vi "WINDOW-System Config.vi"() -> ()   [LabVIEW 2020]
uses:
  User Interface/Windows/System config window/Globals/Sys Config window globals.vi
  User Interface/Windows/System config window/Typedefs/HW config window refs cluster.ctl
  Global Variables/General Globals.vi
  Typedefs/HW config states enum.ctl
  Global Variables/gl_UI Ctrl Refs.vi
  User Interface/Visualisation/Functional Imaging Viewer/Typedefs/Get-Set-Clear Control.ctl
  <vilib>/userDefined/High Color/nirio_resource_hc.ctl
  Typedefs/FPGA input type AC-DC.ctl
  User Interface/Windows/System config window/Typedefs/HW Setup tab control.ctl
  Peripherals Control/Triggers/Typedefs/Trigger setup element cluster.ctl
  Peripherals Control/Triggers/Typedefs/Triggers output setup.ctl
  Typedefs/CTRL system config cluster.ctl
  Typedefs/AOL Properties Cluster.ctl
  RIG-SPECIFIC FILES/FPGA Refs/FPGA Ref.ctl
  Typedefs/DAQ FPGA config cluster.ctl
  Typedefs/Trigger 1 selector enum.ctl
  Peripherals Control/Triggers/Typedefs/General trigger settings cluster.ctl
  Typedefs/Laser 1 config cluster.ctl
  Typedefs/PreChirper 1 config cluster.ctl
  Typedefs/Encoder config cluster.ctl
  Typedefs/Laser Power Control HW config.ctl
  Typedefs/Cam VidRec HW config setup cluster.ctl
  Typedefs/Triggers HW config.ctl
  Typedefs/Objective Config.ctl
  Typedefs/AOD Settings-distilled.ctl
  Typedefs/Prechirper Cal Config.ctl
  Typedefs/PreChirper constants.ctl
  Typedefs/CTRL system config.ctl
  Typedefs/Control Sys HW config cluster.ctl
  Typedefs/DAQ FPGA HW config cluster.ctl
  Typedefs/DAQ FPGA system config.ctl
  Typedefs/Comms Type.ctl
  Typedefs/Peripherals comms config cluster.ctl
  Peripherals Control/XYZ Stage/Control/typedefs/XYZControlConfig.ctl
panel:
  in  "Y stage available":bool
  in  "Y Comms Config Cluster":T1
  in  "DAQ FPGA config cluster":T3={"Target"="RIO0", "input card type"=enum."AC Card", "Ref"=refnum, "Clock Freq (MHz) "=200.0, "Samples Wait after Trigger"=5080, "AOD fill"=4900, "StartupDelay"=0, "Slip Cycle (clock cycles)"=600000, "Add Cycle"=TRUE}
  in  "Control system":T7={"Contrl Sys Available Ind"=FALSE, "Control system.FPGA Type"=enum."Virtex 5", "Control system.Network adapter name"="", "Control system.MAC address"="", "Control system.Ethernet Port"=3, "Ethernet opened"=FALSE, "Ctrl FPGA Clock (MHz)"=240.0, "AOD 1 Amplitude"=0, "AOD 2 Amplitude"=0, "AOD 3 Amplitude"=0, "AOD 4 Amplitude"=0, "AOD 5 Amplitude"=0, "AOD 6 Amplitude"=0, "Data Time Interval (ns)"=0.0, "T0 (ns)"=0.0, "Ta (ns)"=0.0} {"Control system.Ethernet Port" min=0 max=2048 step=1; "Ctrl FPGA Clock (MHz)" min=80.0 max=500.0 step=1.0; "Data Time Interval (ns)" min=0.0 max=2048.0 step=1.0; "Ta (ns)" min=0.0 max=2048.0 step=1.0; "T0 (ns)" min=0.0 max=2048.0 step=1.0; "AOD 6 Amplitude" min=0 max=2048 step=1; "AOD 5 Amplitude" min=0 max=2048 step=1; "AOD 4 Amplitude" min=0 max=2048 step=1; "AOD 3 Amplitude" min=0 max=2048 step=1; "AOD 2 Amplitude" min=0 max=2048 step=1; "AOD 1 Amplitude" min=0 max=2048 step=1}
  in  "Cancel":bool
  in  "OK":bool
  in  "AOL Properties":T8={"AOD 1 thickness (mm)"=118.0, "AOD 2 thickness (mm)"=115.0, "AOD 3 thickness (mm)"=110.0, "AOD 4 thickness (mm)"=135.0, "AOD 5 thickness (mm)"=135.0, "AOD 6 thickness (mm)"=135.0, "AOD 1-2 separation (mm)"=15.0, "AOD 2-3 separation (mm)"=15.0, "AOD 3-4 separation (mm)"=15.0, "AOD 4-5 separation (mm)"=15.0, "AOD 5-6 separation (mm)"=15.0, "AOD 1 X Offset"=15.0, "AOD 2 X Offset"=1.0, "AOD 3 X Offset"=1.0, "AOD 4 X Offset"=1.0, "AOD 1 Y Offset"=1.0, "AOD 2 Y Offset"=1.0, "AOD 3 Y Offset"=1.0, "AOD 4 Y Offset"=1.0, "AOD 1 X Direction"=0.0, "AOD 2 X Direction"=0.0, "AOD 3 X Direction"=0.0, "AOD 4 X Direction"=0.0, "AOD 1 Y Direction"=1.0, "AOD 2 Y Direction"=0.0, "AOD 3 Y Direction"=0.0023, "AOD 4 Y Direction"=0.0046, "AOD 1 Centre (mm)"=15.0, "AOD 2 Centre (mm)"=50.0, "AOD 3 Centre (mm)"=50.0, "AOD 4 Centre (mm)"=50.0, "Timing Offset AOD 1"=0.0, "Timing Offset AOD 2"=0.0, "Timing Offset AOD 3"=0.0, "Timing Offset AOD 4"=0.0, "AOD Optical offset 1"=20000.0, "AOD Optical offset 2"=20000.0, "AOL aperture (mm)"=15.0, "AOL centre wavelength (nm)"=1.0, "AOL centre frequency (MHz)"=1.0, "Diffraction mode"=1.0, "Crystal length (mm)"=0.0, "Acoustic velocity (m/s)"=1.0, "Pair deflection ratio"=1.0, "AOD fill time (us)"=1.0, "AOD Ord. Refractive index"=2.22, "AOD ExtraOrd. Refractive index"=2.22}
  in  "Config Tab Control":T9=enum."Hardware Setup"
  in  "Control Sys. HW config":T10
  in  "Controller System Config":T11={"AOD 1 Amplitude"=0, "AOD 2 Amplitude"=0, "AOD 3 Amplitude"=0, "AOD 4 Amplitude"=0, "AOD 5 Amplitude"=0, "AOD 6 Amplitude"=0, "T0 (ns)"=0.0, "Ta (ns)"=0.0, "Data Time Interval (ns)"=0.0, "Ctrl FPGA Clock (MHz)"=240.0} {"Ctrl FPGA Clock (MHz)" min=80.0 max=500.0 step=1.0; "Data Time Interval (ns)" min=0.0 max=2048.0 step=1.0; "Ta (ns)" min=0.0 max=2048.0 step=1.0; "T0 (ns)" min=0.0 max=2048.0 step=1.0; "AOD 6 Amplitude" min=0 max=2048 step=1; "AOD 5 Amplitude" min=0 max=2048 step=1; "AOD 4 Amplitude" min=0 max=2048 step=1; "AOD 3 Amplitude" min=0 max=2048 step=1; "AOD 2 Amplitude" min=0 max=2048 step=1; "AOD 1 Amplitude" min=0 max=2048 step=1}
  in  "Ctrl FPGA available":bool
  in  "DAQ FPGA System Config":T12={"Clock Freq (MHz) "=200.0, "Samples Wait after Trigger"=5080, "AOD fill"=4900, "StartupDelay"=0, "Slip Cycle (clock cycles)"=600000, "Add Cycle"=TRUE}
  in  "DAQ FPGA HW Config":T13={"FGPA Ref"=refnum, "Target"="RIO0", "input card type"=enum."AC Card"}
  in  "Triggers sub-tab control":enum32{"General", "Routing & Timing"}(tab)
  in  "Trigger HW config":T14
  in  "General trigger settings":T15={"Trigger 1 function"=enum."Encoder trigger", "Triggers loop clock (MHz)"=80.0} {"Triggers loop clock (MHz)" format="%#_13g"}
  in  "Triggers output setup":T17 {"Pulse width (us)" min=10 max=5000 step=1 format="%.0fµs"}
  in  "Externalise Triggers":bool
  in  "PMT Voltage Upper Limit":dbl
  in  "PMT Voltage Lower Limit":dbl
  in  "Galvo AOs":tag
  in  "Power meter AI":tag
  in  "Pockels AO":tag
  in  "PMT AOs":tag
  in  "Hard shutter AO":tag
  in  "Z Comms Config Cluster":T1
  in  "XY Comms Config Cluster":T1
  in  "Z stage available":bool
  in  "XY stage available":bool
  in  "XYZ Stage Control Config":T19
  in  "Encoder":T20={"IP address"="224.0.1.103", "Port"=7000, "Wheel radius (cm)"=16.0, "Encoder Trigger"=""} {"Wheel radius (cm)" format="%#_13g"}
  in  "Wheel radius (cm)":dbl format="%#_13g"
  in  "Encoder IP address":string="224.0.1.103"
  in  "Encoder port":u16=7000
  in  "Encoder available":bool
  in  "Axial MC Supported":bool caption="Axial Movement Correction Supported"
  in  "MC Supported":bool caption="Movement Correction Supported"
  in  "Computer MAC address":string="82574L"
  in  "Demo mode":enum16{"Full functionality", "Demo mode"}(ring) caption="Mode"
  in  "Number of AODs":dbl=4.0
  in  "Swap XY on stage":bool
  in  "DO flag-Trial start":tag
  in  "DO flag-Video record":tag
  in  "Cam VidRec available":bool caption="Cameras video recording system is available"
  in  "Cam VidRec":T21
  in  "AOD Settings - distilled":T22={"AOD 1 thickness (mm)"=8.0, "AOD 2 thickness (mm)"=8.0, "AOD 3 thickness (mm)"=8.0, "AOD 4 thickness (mm)"=8.0, "AOD 1-2 separation (mm)"=50.0, "AOD 2-3 separation (mm)"=50.0, "AOD 3-4 separation (mm)"=50.0, "AOD 1 Centre (mm)"=7.5, "AOD 2 Centre (mm)"=7.5, "AOD 3 Centre (mm)"=7.5, "AOD 4 Centre (mm)"=7.5, "AOD 1 X Offset"=0.0, "AOD 2 X Offset"=0.0023, "AOD 3 X Offset"=0.0046, "AOD 4 X Offset"=0.0046, "AOD 1 Y Offset"=0.0, "AOD 2 Y Offset"=0.0, "AOD 3 Y Offset"=0.0023, "AOD 4 Y Offset"=0.0046, "Timing Offset AOD 1"=0.0, "Timing Offset AOD 2"=0.0, "Timing Offset AOD 3"=0.0, "Timing Offset AOD 4"=0.0, "AOL centre wavelength (nm)"=1.0, "AOL centre frequency (MHz)"=1.0, "Pair deflection ratio"=1.0, "AOL aperture (mm)"=15.0, "AOD fill time (us)"=1.0, "Diffraction mode"=1.0, "Crystal length (mm)"=0.0, "Acoustic velocity (m/s)"=1.0, "AOD Ord. Refractive index"=2.22}
  in  "Current Objective":string
  in  "Objective Calibration Settings":T23[](array[typedef])
  in  "Pockels cal.Dwell time (µs)":dbl=0.4 caption="Dwell time (µs)" min=0.05 max=12.0 step=0.1 format="%#.2fµs"
  in  "Pockels cal.Zoom":u8=12 caption="Zoom" min=1 max=24 step=1 format="x%.0f"
  in  "Laser 1 available":bool
  in  "Laser 1 config":T24={"COM port"="COM7", "Baud Rate"=0, "Type"=""}
  in  "Laser Power Control HW config":T25={"Laser Power Control"="Pockels", "Laser Power Modulation Control"=enum."NI"}
  in  "Laser Wavelength 2":u16(ring) caption="Laser Wavelength (nm)" items=["920"]
  in  "Prechirper 1 available":bool
  in  "Prechirper 1 config":T26={"Type"="", "Baud Rate"=0, "COM port"="COM7"}
  in  "PreChirper Preset Calibration Values":T27[](array[typedef])
  in  "Prechirper Constants":T28
  in  "PreChirp Preset Values":bool caption="Use Preset Values"
  in  "Initial Laser Wavelength [nm]":dbl=5.0
  in  "Initial Dwell Time [us]":dbl=5.0
  in  "Error Logging":bool
  in  "Performance Monitoring":bool caption="PC Performance Monitoring"
  in  "Microscope ID":string="003"
  in  "Microscope Type":string="AOLM"
  in  "Revision Number":string="1.0.0.0"
  in  "Advanced Imaging":bool
  in  "Max Allowed Trial Length [s]":dbl=60.0
  in  "Initial Scan Resolution":dbl=512.0
  in  "Initial Acceptance Angle [mrad]":dbl=5.0
  # "This functionality connects the various PXI backplane triggers to physical terminals on the DI/O module.\n\n\nOriginal setup:\nPXI_Trigger 0= Unused\nPXI_Trigger 1= Line trigger\nPXI_Trigger 2= Frame trigger / Cycle trigge\nPXI_Trigger 3= Trial trigger\nPXI_Trigger 4= Start of Experiment trigger\nPXI_Trigger 5= Stimulus trigger"
  # "(make , model etc)"
  # "(COM Port / IP Address / service address etc.)"
  # "(Port for ethernet / channel for BT)"
  # "[HWC]"
  # "[DNT]"
  # "NOTE: The triggers setup is part of the user-profiles functionality.\nSave the current user profile to retain any changes you make above.\nChanges will not be automatically saved."
  # "'Externalise Triggers' must be enabled"
  # "[DNT]"
  # "[HWC]"
  # "(make , model etc)"
  # "(COM Port / IP Address / service address etc.)"
  # "(Port for ethernet / channel for BT)"
  # "(make , model etc)"
  # "(COM Port / IP Address / service address etc.)"
  # "(Port for ethernet / channel for BT)"
  # "[Delete me later]"
  # "Thickness (mm)"
  # "X Offset"
  # "Separation (mm)"
  # "Y Offset"
  # "Centre (mm)"
  # "Timing Offset"
  # "Pockels Calibration Conditions"
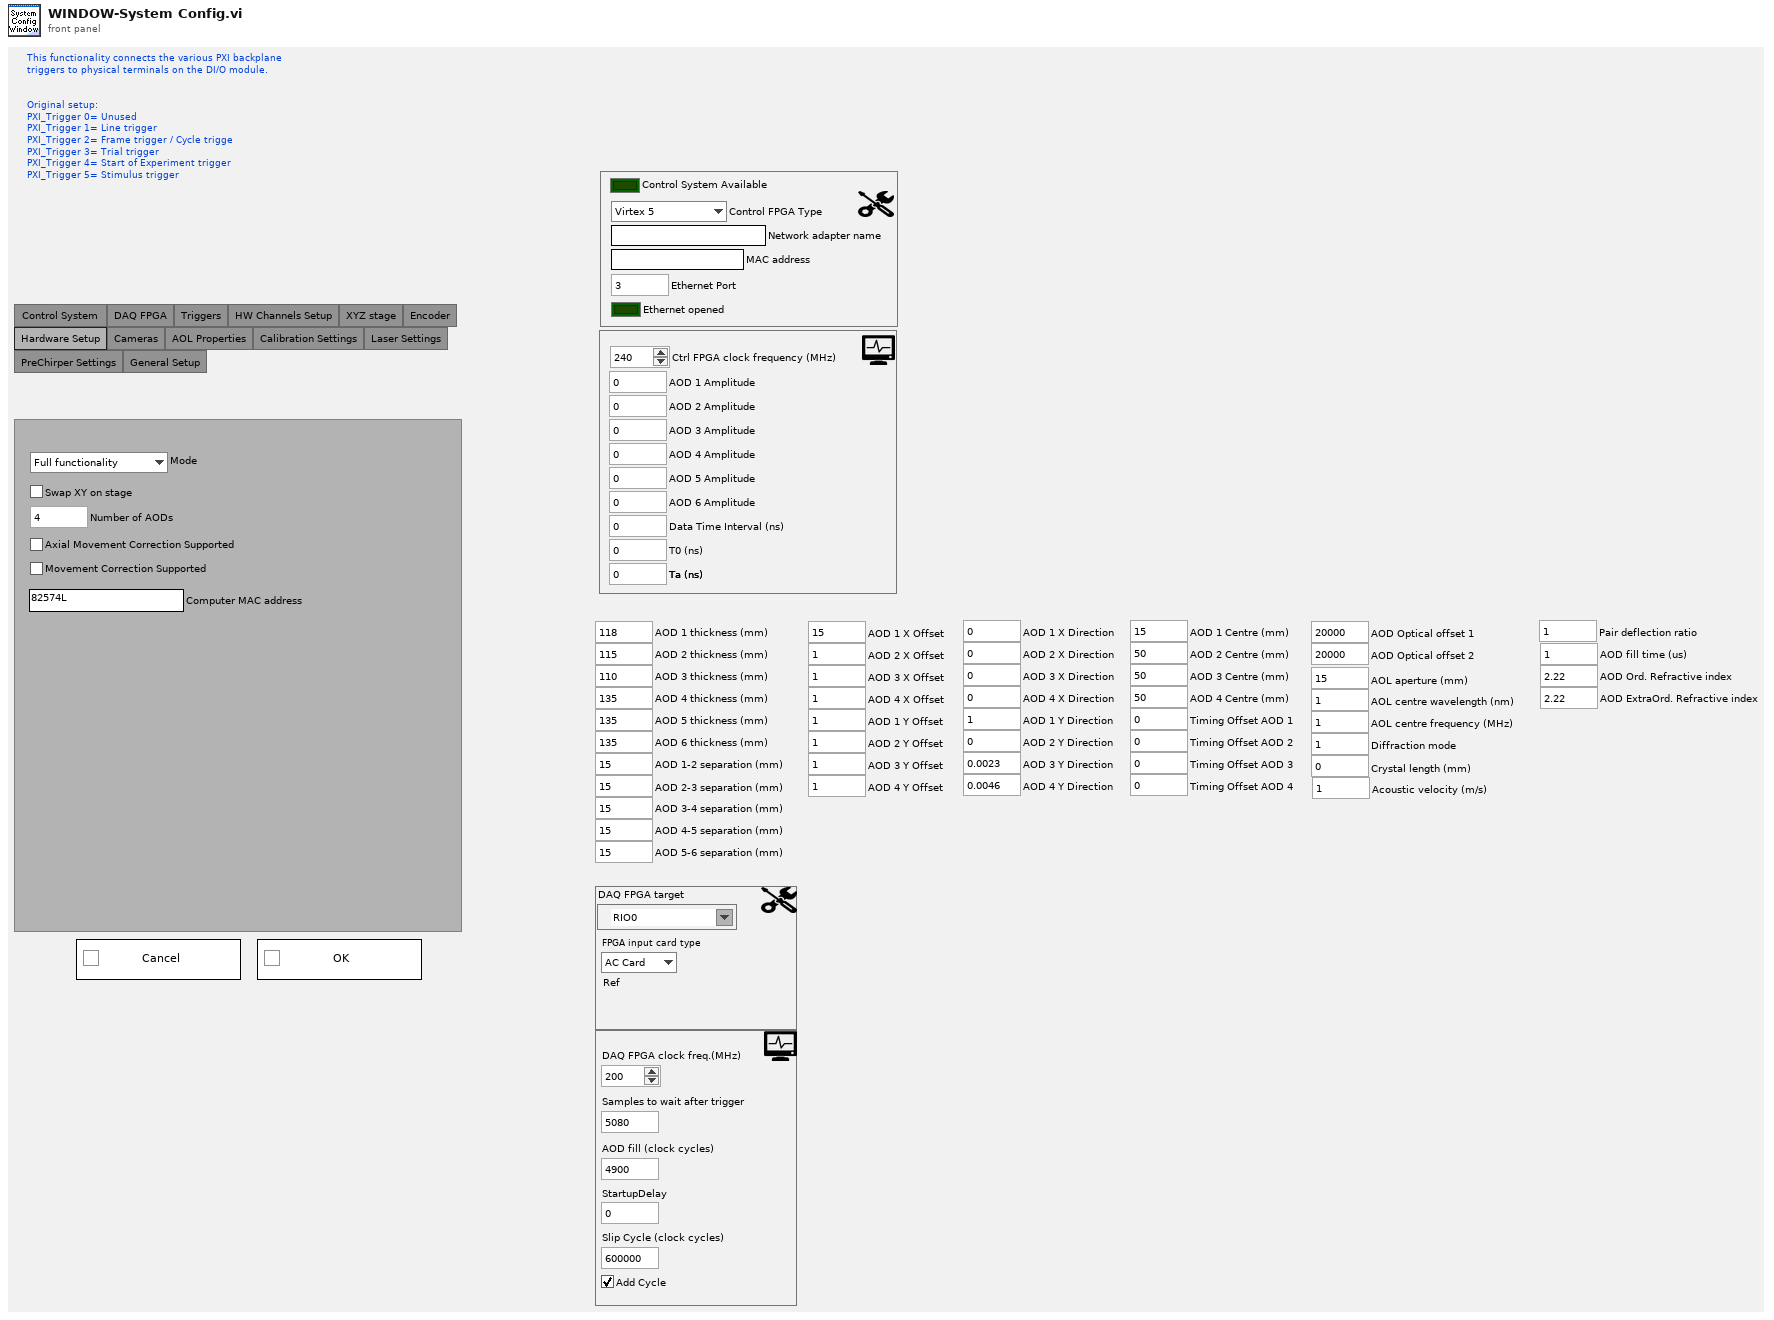
[diagram p1: front panel]
types:
  T1 = typedef "Peripherals comms config cluster.ctl" = cluster{"Name":string, "Device Address":string, "Port ":u16, "Baudrate":i32, "Comms Type":T2}
  T2 = typedef "Comms Type.ctl" = enum16{"GPIB-IEEE488", "Serial-RS232", "Serial-RS485", "Serial-RS422", "Serial-USB", "Ethernet-TCP/IP", "Ethernet-UDP"}
  T3 = typedef "DAQ FPGA config cluster.ctl" = cluster{"Target":T4, "input card type":T5, "Ref":T6, "Clock Freq (MHz) ":dbl, "Samples Wait after Trigger":u16, "AOD fill":u16, "StartupDelay":i32, "Slip Cycle (clock cycles)":u32, "Add Cycle":bool}
  T4 = typedef "nirio_resource_hc.ctl" = tag
  T5 = typedef "FPGA input type AC-DC.ctl" = enum16{"AC Card", "DC Card"}
  T6 = typedef "FPGA Ref.ctl" = refnum<k20>
  T7 = typedef "CTRL system config cluster.ctl" = cluster{"Contrl Sys Available Ind":bool, "Control system.FPGA Type":enum16{"Virtex 5", "Virtex 7"}, "Control system.Network adapter name":string, "Control system.MAC address":string, "Control system.Ethernet Port":i16, "Ethernet opened":bool, "Ctrl FPGA Clock (MHz)":dbl, "AOD 1 Amplitude":i16, "AOD 2 Amplitude":i16, "AOD 3 Amplitude":i16, "AOD 4 Amplitude":i16, "AOD 5 Amplitude":i16, "AOD 6 Amplitude":i16, "Data Time Interval (ns)":dbl, "T0 (ns)":dbl, "Ta (ns)":dbl}
  T8 = typedef "AOL Properties Cluster.ctl" = cluster{"AOD 1 thickness (mm)":dbl, "AOD 2 thickness (mm)":dbl, "AOD 3 thickness (mm)":dbl, "AOD 4 thickness (mm)":dbl, "AOD 5 thickness (mm)":dbl, "AOD 6 thickness (mm)":dbl, "AOD 1-2 separation (mm)":dbl, "AOD 2-3 separation (mm)":dbl, "AOD 3-4 separation (mm)":dbl, "AOD 4-5 separation (mm)":dbl, "AOD 5-6 separation (mm)":dbl, "AOD 1 X Offset":dbl, "AOD 2 X Offset":dbl, "AOD 3 X Offset":dbl, "AOD 4 X Offset":dbl, "AOD 1 Y Offset":dbl, "AOD 2 Y Offset":dbl, "AOD 3 Y Offset":dbl, "AOD 4 Y Offset":dbl, "AOD 1 X Direction":dbl, "AOD 2 X Direction":dbl, "AOD 3 X Direction":dbl, "AOD 4 X Direction":dbl, "AOD 1 Y Direction":dbl, "AOD 2 Y Direction":dbl, "AOD 3 Y Direction":dbl, "AOD 4 Y Direction":dbl, "AOD 1 Centre (mm)":dbl, "AOD 2 Centre (mm)":dbl, "AOD 3 Centre (mm)":dbl, "AOD 4 Centre (mm)":dbl, "Timing Offset AOD 1":dbl, "Timing Offset AOD 2":dbl, "Timing Offset AOD 3":dbl, "Timing Offset AOD 4":dbl, "AOD Optical offset 1":dbl, "AOD Optical offset 2":dbl, "AOL aperture (mm)":dbl, "AOL centre wavelength (nm)":dbl, "AOL centre frequency (MHz)":dbl, "Diffraction mode":dbl, "Crystal length (mm)":dbl, "Acoustic velocity (m/s)":dbl, "Pair deflection ratio":dbl, "AOD fill time (us)":dbl, "AOD Ord. Refractive index":dbl, "AOD ExtraOrd. Refractive index":dbl}
  T9 = typedef "HW Setup tab control.ctl" = enum32{"Control System ", "DAQ FPGA", "Triggers", "HW Channels Setup", "XYZ stage", "Encoder", "Hardware Setup", "Cameras", "AOL Properties", "Calibration Settings", "Laser Settings", "PreChirper Settings", "General Setup"}
  T10 = typedef "Control Sys HW config cluster.ctl" = cluster{"Control system.FPGA Type":enum16{"Virtex 5", "Virtex 7"}, "Control system.Network adapter name":string, "Control system.MAC address":string, "Control system.Ethernet Port":u32, "Control system.Ethernet Port Opened":bool}
  T11 = typedef "CTRL system config.ctl" = cluster{"AOD 1 Amplitude":i16, "AOD 2 Amplitude":i16, "AOD 3 Amplitude":i16, "AOD 4 Amplitude":i16, "AOD 5 Amplitude":i16, "AOD 6 Amplitude":i16, "T0 (ns)":dbl, "Ta (ns)":dbl, "Data Time Interval (ns)":dbl, "Ctrl FPGA Clock (MHz)":dbl}
  T12 = typedef "DAQ FPGA system config.ctl" = cluster{"Clock Freq (MHz) ":dbl, "Samples Wait after Trigger":u16, "AOD fill":u16, "StartupDelay":i32, "Slip Cycle (clock cycles)":u32, "Add Cycle":bool}
  T13 = typedef "DAQ FPGA HW config cluster.ctl" = cluster{"FGPA Ref":T6, "Target":T4, "input card type":T5}
  T14 = typedef "Triggers HW config.ctl" = cluster{"Available Device List":i32, "Device Address":string}
  T15 = typedef "General trigger settings cluster.ctl" = cluster{"Trigger 1 function":T16, "Triggers loop clock (MHz)":dbl}
  T16 = typedef "Trigger 1 selector enum.ctl" = enum16{"Encoder trigger", "Line trigger", "Control system's ref frame acknowledgement"}
  T17 = typedef "Triggers output setup.ctl" = T18[]
  T18 = typedef "Trigger setup element cluster.ctl" = cluster{"Name":string, "Output?":bool, "Output terminal":tag, "PXI backplane line":tag, "Pulse width (us)":u16}
  T19 = typedef "XYZControlConfig.ctl" = enum16{"None", "XYZ", "XY-Z", "X-Y-Z", "Z"}
  T20 = typedef "Encoder config cluster.ctl" = cluster{"IP address":string, "Port":u16, "Wheel radius (cm)":dbl, "Encoder Trigger":tag}
  T21 = typedef "Cam VidRec HW config setup cluster.ctl" = cluster{"DO flag-Video record":tag, "DO flag-Trial start":tag}
  T22 = typedef "AOD Settings-distilled.ctl" = cluster{"AOD 1 thickness (mm)":dbl, "AOD 2 thickness (mm)":dbl, "AOD 3 thickness (mm)":dbl, "AOD 4 thickness (mm)":dbl, "AOD 1-2 separation (mm)":dbl, "AOD 2-3 separation (mm)":dbl, "AOD 3-4 separation (mm)":dbl, "AOD 1 Centre (mm)":dbl, "AOD 2 Centre (mm)":dbl, "AOD 3 Centre (mm)":dbl, "AOD 4 Centre (mm)":dbl, "AOD 1 X Offset":dbl, "AOD 2 X Offset":dbl, "AOD 3 X Offset":dbl, "AOD 4 X Offset":dbl, "AOD 1 Y Offset":dbl, "AOD 2 Y Offset":dbl, "AOD 3 Y Offset":dbl, "AOD 4 Y Offset":dbl, "Timing Offset AOD 1":dbl, "Timing Offset AOD 2":dbl, "Timing Offset AOD 3":dbl, "Timing Offset AOD 4":dbl, "AOL centre wavelength (nm)":dbl, "AOL centre frequency (MHz)":dbl, "Pair deflection ratio":dbl, "AOL aperture (mm)":dbl, "AOD fill time (us)":dbl, "Diffraction mode":dbl, "Crystal length (mm)":dbl, "Acoustic velocity (m/s)":dbl, "AOD Ord. Refractive index":dbl}
  T23 = typedef "Objective Config.ctl" = cluster{"Name":string, "Sum X":dbl, "Sum Y":dbl, "Diff X":dbl, "Diff Y":dbl, "Distortion Correction":dbl, "Z_norm to um_scaling":dbl, "X_norm to um_scaling":dbl, "Calibrated Wavelength":dbl}
  T24 = typedef "Laser 1 config cluster.ctl" = cluster{"COM port":refnum<visa-resource-name>, "Baud Rate":i32, "Type":string}
  T25 = typedef "Laser Power Control HW config.ctl" = cluster{"Laser Power Control":string, "Laser Power Modulation Control":enum16{"NI", "FPGA"}}
  T26 = typedef "PreChirper 1 config cluster.ctl" = cluster{"Type":string, "Baud Rate":i32, "COM port":refnum<visa-resource-name>}
  T27 = typedef "Prechirper Cal Config.ctl" = cluster{"Wavelength":i32, "Prism 1":i32, "Prism 2":i32}
  T28 = typedef "PreChirper constants.ctl" = cluster{"a 1":i32, "b 1":i32, "c 1":i32, "a 2":i32, "b 2":i32, "c 2":i32, "lmin":i32, "lmax":i32}
  T29 = typedef "HW config window refs cluster.ctl" = cluster{"VI's reference":refnum<vi>, "menu reference":refnum<k9>, "Pane":refnum<vi>, "Config Tab Control":refnum<vi>, "Triggers sub-tab control":refnum<vi>, "Microscope ID":refnum<vi>, "Microscope Type":refnum<vi>, "Revision Number":refnum<vi>, "Advanced Imaging":refnum<vi>, "Max Allowed Trial Length":refnum<vi>, "Initial Scan Resolution":refnum<vi>, "Initial Acceptance Angle":refnum<vi>, "Initial Laser Wavelength [nm] ":refnum<vi>, "Initial Dwell Time [us]":refnum<vi>, "Error Logging":refnum<vi>, "Performance Monitoring":refnum<vi>, "Ctrl FPGA available":refnum<vi>, "Control HW config":refnum<vi>, "Control System Config":refnum<vi>, "General trigger settings":refnum<vi>, "Trigger HW config":refnum<vi>, "Externalise Triggers":refnum<vi>, "[Triggers output setup]":refnum<vi>, "DAQ FPGA HW Config":refnum<vi>, "DAQ FPGA System Config":refnum<vi>, "Pockels AO":refnum<vi>, "Hard shutter AO":refnum<vi>, "PMT AOs":refnum<vi>, "Galvo AO":refnum<vi>, "Power meter AI":refnum<vi>, "PMT Voltage Lower Limit":refnum<vi>, "PMT Voltage Upper Limit":refnum<vi>, "XYZ Stage Control Config":refnum<vi>, "XY stage available":refnum<vi>, "XY Comms Config Cluster":refnum<vi>, "Y stage available":refnum<vi>, "Y Comms Config Cluster":refnum<vi>, "Z stage available":refnum<vi>, "Z Comms Config Cluster":refnum<vi>, "Encoder available":refnum<vi>, "Encoder":refnum<vi>, "Encoder IP address":refnum<vi>, "Encoder port":refnum<vi>, "Wheel radius (cm)":refnum<vi>, "Demo mode":refnum<vi>, "Swap XY on stage":refnum<vi>, "Number of AODs":refnum<vi>, "Axial MC Supported":refnum<vi>, "MC Supported":refnum<vi>, "Computer MAC add.":refnum<vi>, "Cam VidRec available":refnum<vi>, "Cam VidRec":refnum<vi>, "DO flag-Video record":refnum<vi>, "DO flag-Trial start":refnum<vi>, "AOD Settings (distilled)":refnum<vi>, "Pockels cal.Dwell time (µs)":refnum<vi>, "Pockels cal.Zoom":refnum<vi>, "Current Objective":refnum<vi>, "[Obj. Calib. Settings]":refnum<vi>, "Laser Wavelength":refnum<vi>, "Laser Power Control \nHW config":refnum<vi>, "Laser 1 available":refnum<vi>, "Laser 1 config":refnum<vi>, "Prechirper 1 available":refnum<vi>, "Prechirper 1 config":refnum<vi>, "PreChirp Preset Values":refnum<vi>, "[PreChirper Preset \nCalibration Values]":refnum<vi>, "Prechirper Constants":refnum<vi>}
  T30 = typedef "Initial config.ctl" = cluster{"Triggers output setup":T17, "General trigger settings":T15, "Calibration settings":T31, "Hardware Configuration":T32, "System Config":T35, "Calibration config.":T36, "General Setup":T37, "AOD Settings - distilled":T22}
  T31 = typedef "Pockels Calibration settings cluster.ctl" = cluster{"Pockels cal.Zoom":u8, "Pockels cal.Dwell time (µs)":dbl}
  T32 = typedef "Hardware Configuration settings.ctl" = cluster{"Dev. PC":bool, "Swap XY on stage":bool, "No of AOD":u8, "MC Supported":bool, "Axial MC":bool, "Computer MAC address":string, "Externalise Triggers":bool, "Trigger HW config":T14, "DAQmx Chan":T33, "XYZ Stage Control Config":T19, "XY stage available":bool, "XY Comms Config Cluster":T1, "Y stage available":bool, "Y Comms Config Cluster":T1, "Z stage available":bool, "Z Comms Config Cluster ":T1, "Encoder available":bool, "Encoder":T20, "VidRec available":bool, "Cam VidRec":T21, "Laser Power Control HW config":T25, "Laser 1 available":bool, "Laser 1 config cluster":T24, "Prechirper 1 available":bool, "Prechirper 1 config cluster":T26, "Control system.FPGA available?":bool, "Control Sys. HW config":T10, "DAQ FPGA HW Config":T13, "PMT Control Voltage Limits":T34}
  T33 = typedef "DAQmx physical channels cluster.ctl" = cluster{"Pockels AO":tag, "Hard shutter AO":tag, "PMT AOs":tag, "Galvo AOs":tag, "Power meter AI":tag}
  T34 = typedef "PMT Control Voltage limits.ctl" = cluster{"Lower Limit":dbl, "Upper Limit":dbl}
  T35 = typedef "System Configuration.ctl" = cluster{"Laser wavelength (nm)":dbl, "DAQ FPGA System":T12, "Control system":T11}
  T36 = typedef "Calibration config.ctl" = cluster{"Current Objective":string, "Objective Settings":T23[], "PreChirper Values Preset ?":bool, "PreChirper Settings":T27[], "PreChirper Constants":T28}
  T37 = typedef "General Setup.ctl" = cluster{"Microscope ID":string, "Microscope Type":string, "Revision Number":string, "Advanced Imaging":bool, "Error Logging":bool, "Performance Monitoring":bool, "Max Allowed Trial Length":dbl, "Initial Scan Resolution":dbl, "Initial Acceptance Angle":dbl, "Initial Laser Wavelength":dbl, "Initial Dwell Time":dbl}
  T38 = enum32{"Invalid", "Standard", "Closed", "Hidden", "Minimized", "Maximized"}
  T39 = typedef "Get-Set-Clear Control.ctl" = enum16{"Get", "Set", "Clear"}
  T40 = typedef "HW config states enum.ctl" = enum16{"Load from file", "Save to file", "Save backup", "Write all", "Read all", "Write XY stage settings", "Write DAQ FPGA settings", "Write Control FPGA settings", "Write Phys Channels", "Write System Config", "Write HW Config", "Save System Config", "Save HW Config", "Clear", "Compare from file"}
  T41 = typedef "UI ctrl refs cluster.ctl" = cluster{"Top level VI path":path, "Top level VI ref":refnum<vi>, "User menu ref":refnum<k9>, "Sub Panel control":refnum<vi>, "Imaging Param Tab":refnum<vi>, "Occurrence-Start drivers":refnum<k4>, "Occurrence-Speed logging initialised":refnum<k4>, "Occurrence-XYZ stage initialised":refnum<k4>, "Exit button":refnum<vi>, "Status ind":refnum<vi>, "Set as origin":refnum<vi>, "Speed Logging":refnum<vi>, "Time Lapse":refnum<vi>, "Live Imaging":refnum<vi>, "AOL Z Stack":refnum<vi>, "Motor Z Stack":refnum<vi>, "Funct Acq button":refnum<vi>, "Hard Shutter":refnum<vi>, "Virtual Shutter":refnum<vi>, "Laser Power":refnum<vi>, "AOL Mode":refnum<vi>, "Frame Size":refnum<vi>, "Field of View":refnum<vi>, "Dwell Time":refnum<vi>, "Zoom":refnum<vi>, "AOL Z":refnum<vi>, "Objective":refnum<vi>, "Axis":refnum<vi>, "Paths & Names":refnum<vi>, "Experiment folder path (ind.)":refnum<vi>, "Last State (Ind.)":refnum<vi>, "Averages":refnum<vi>, "Angle (degrees)":refnum<vi>, "X centre":refnum<vi>, "Y centre":refnum<vi>, "Plane Mode":refnum<vi>, "# Planes":refnum<vi>, "Z Start":refnum<vi>, "Z Stop":refnum<vi>, "Z Step":refnum<vi>, "PMT 1":refnum<vi>, "PMT 2":refnum<vi>, "Stage XYZ Position":refnum<vi>, "Pockels@Z Start":refnum<vi>, "Pockels@Z Stop":refnum<vi>, "Obtain Z Start":refnum<vi>, "Obtain Z Stop":refnum<vi>, "Live stim.trig.period":refnum<vi>, "Live stim.trig.enable":refnum<vi>, "Movement Correction":refnum<vi>, "Load Reference Image":refnum<vi>, "XY Stage Move":refnum<vi>, "MovCor Cluster":refnum<vi>, "RefDAQParam":refnum<vi>, "Funct. Acq. Pockels Modulation":refnum<vi>, "Ref Laser Power":refnum<vi>, "Enable Video Recording":refnum<vi>, "Video Record-Live Imaging":refnum<vi>, "Video Record-Funct acq":refnum<vi>, "Reference Source":refnum<vi>, "AOL Z-stack Chirps Ready (ind)":refnum<vi>, "Target time between mov.cor. ref triggers (ms)":refnum<vi>, "Funct. Acq. Ref frame save":refnum<vi>, "Tracking button":refnum<vi>, "Show ref plots window":refnum<vi>, "Center freq ind (nm)":refnum<vi>, "Pickup mode (ind)":refnum<vi>, "Logging queue (ind)":refnum<vi>, "Back aperture power (ind.)":refnum<vi>, "Power after objective (ind.)":refnum<vi>, "Switch user":refnum<vi>, "Ls1 Conn. Status":refnum<vi>, "Ls1Tuning Status":refnum<vi>, "Ls1 Faults":refnum<vi>, "Ls1 Connection":refnum<vi>, "Ls1 Mode":refnum<vi>, "Ls1 POWER [mW]":refnum<vi>, "Ls1Shutter":refnum<vi>, "Ls1 Wavelength":refnum<vi>, "Ls1 Note":refnum<vi>, "Ls1 Confirm Wav":refnum<vi>, "Ls1 PreChrp Prism1":refnum<vi>, "Ls1 PreChrp Prism2":refnum<vi>, "Ls1 wav top Ind":refnum<vi>, "Ls1 power top Ind":refnum<vi>, "Ls1 Pump peak Hold":refnum<vi>, "Ls1 Status Ind":refnum<vi>, "Ls1 wav cancel":refnum<vi>, "Experiment Type":refnum<vi>, "Biology Information":refnum<vi>, "Camera recording status":refnum<vi>, "Optimise Obj. Pos.":refnum<vi>}
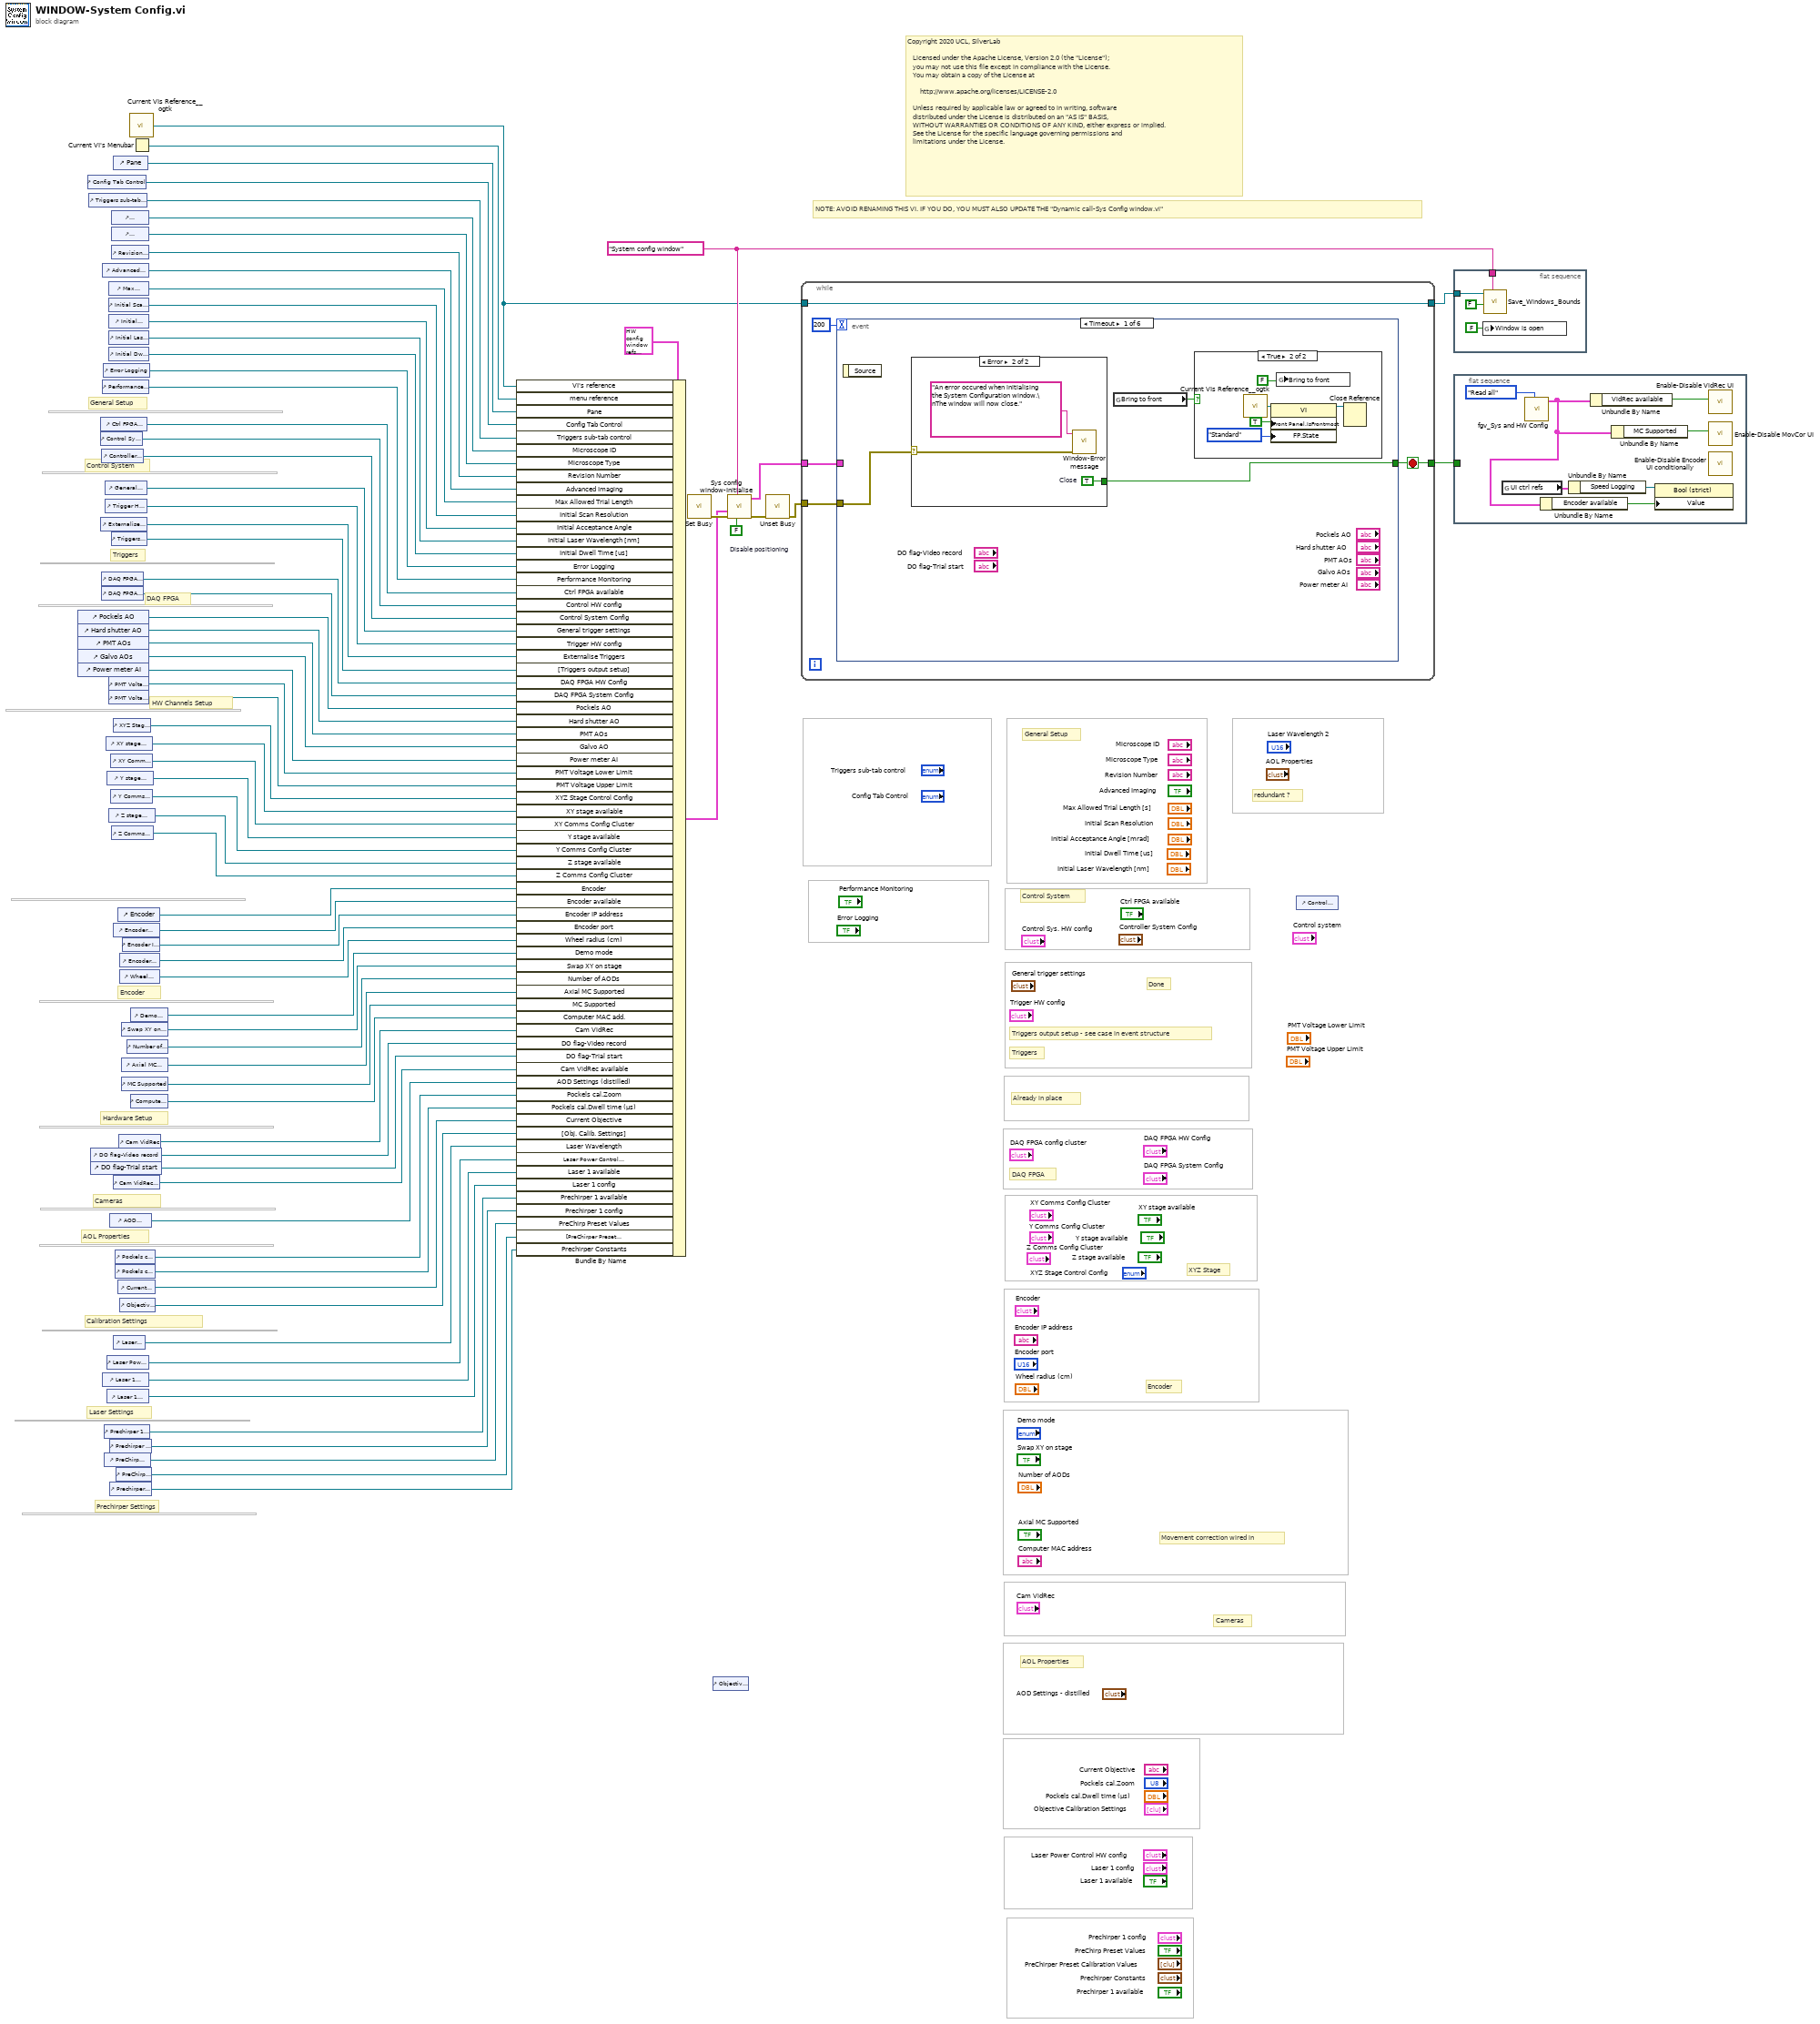
[diagram p0: block diagram]
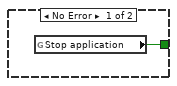
[diagram p3: hidden frame]
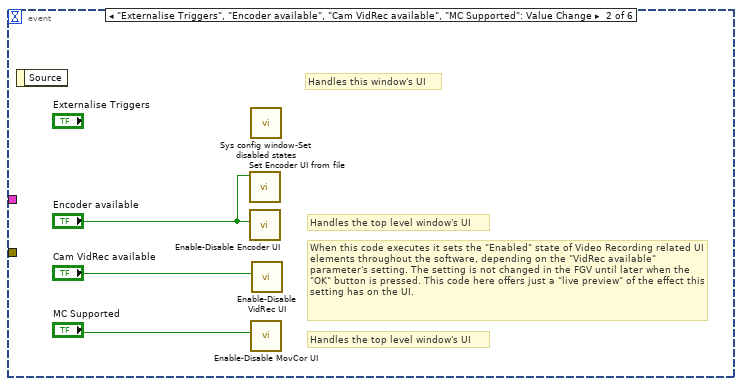
[diagram p4: hidden frame]
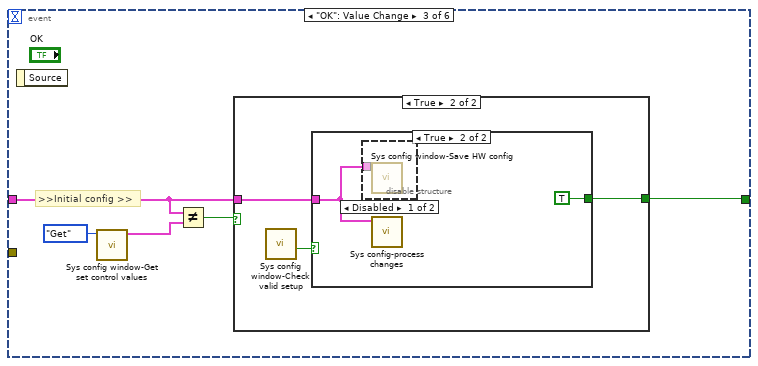
[diagram p5: hidden frame]
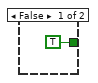
[diagram p6: hidden frame]
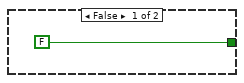
[diagram p7: hidden frame]
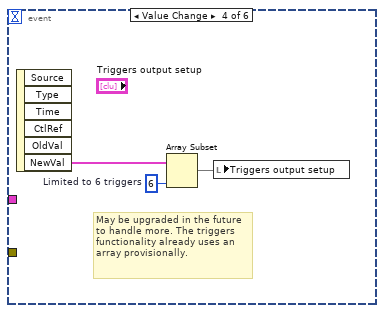
[diagram p9: hidden frame]
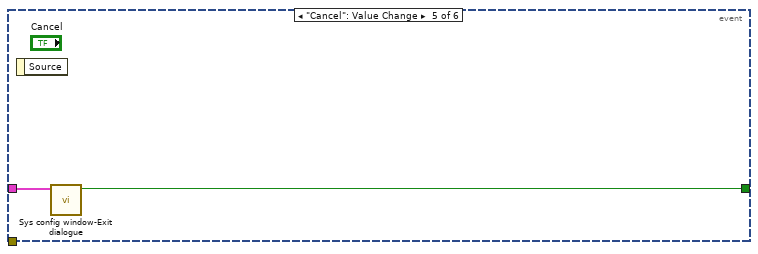
[diagram p10: hidden frame]
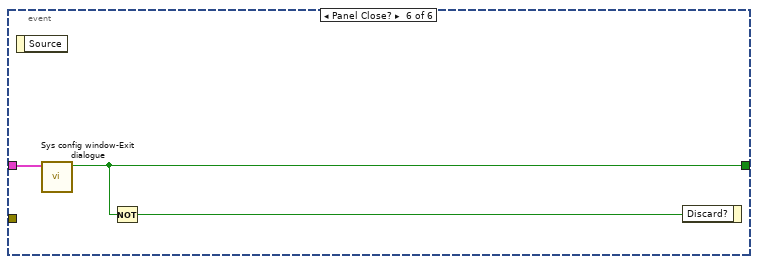
[diagram p11: hidden frame]
diagram:
  w68 = FALSE  # Disable positioning
  w69 = "System config window" ("Window Name (i.e. Key)")
  # "Copyright 2020 UCL, SilverLab\n \n   Licensed under the Apache License, Version 2.0 (the \"License\");\n   you may not use this file except in compliance with the License.\n   You may obtain a copy of the License at\n \n       http://www.apache.org/licenses/LICENSE-2.0\n \n   Unless required by applicable law or agreed to in writing, software\n   distributed under the License is distributed on an \"AS IS\" BASIS,\n   WITHOUT WARRANTIES OR CONDITIONS OF ANY KIND, either express or implied.\n   See the License for the specific language governing permissions and\n   limitations under the License."
  # "Prechirper Settings"
  # "Laser Settings"
  # "Calibration Settings"
  # "AOL Properties"
  # "Cameras"
  # "Hardware Setup"
  # "Encoder"
  # "HW Channels Setup"
  # "DAQ FPGA"
  # "Triggers"
  # "Control System"
  # "General Setup"
  # "Done"
  # "redundant ?"
  # "AOL Properties"
  # "Cameras"
  # "Movement correction wired in"
  # "Encoder"
  # "Already in place"
  # "XYZ Stage"
  # "DAQ FPGA"
  # "Triggers output setup - see case in event structure"
  # "Triggers"
  # "Control System"
  # "General Setup"
  # "NOTE: AVOID RENAMING THIS VI. IF YOU DO, YOU MUST ALSO UPDATE THE \"Dynamic call-Sys Config window.vi\""
  n1 = control-ref of="Pockels AO"() -> (w52:refnum<vi>)
  n2 = control-ref of="Hard shutter AO"() -> (w51:refnum<vi>)
  n3 = control-ref of="PMT AOs"() -> (w50:refnum<vi>)
  n4 = control-ref of="Galvo AOs"() -> (w49:refnum<vi>)
  n5 = control-ref of="Power meter AI"() -> (w48:refnum<vi>)
  n6 = control-ref of="Config Tab Control"() -> (w21:refnum<vi>)
  n7 = control-ref of="Triggers sub-tab control"() -> (w63:refnum<vi>)
  n8 = control-ref of="DO flag-Video record"() -> (w71:refnum<vi>)
  n9 = control-ref of="DO flag-Trial start"() -> (w70:refnum<vi>)
  n10 = control-ref of="Ctrl FPGA available"() -> (w20:refnum<vi>)
  n11 = control-ref of="Control Sys. HW config"() -> (w12:refnum<vi>)
  n12 = control-ref of="Externalise Triggers"() -> (w53:refnum<vi>)
  n13 = control-ref of="Controller System Config"() -> (w11:refnum<vi>)
  n14 = control-ref of="DAQ FPGA HW Config"() -> (w10:refnum<vi>)
  n15 = control-ref of="DAQ FPGA System Config"() -> (w9:refnum<vi>)
  n16 = control-ref of="Advanced Imaging"() -> (w59:refnum<vi>)
  n17 = control-ref of="Performance Monitoring"() -> (w13:refnum<vi>)
  n18 = control-ref of="Laser 1 available"() -> (w18:refnum<vi>)
  n19 = control-ref of="Error Logging"() -> (w14:refnum<vi>)
  n20 = control-ref of="Prechirper 1 available"() -> (w17:refnum<vi>)
  n21 = control-ref of="PreChirp Preset Values"() -> (w25:refnum<vi>)
  n22 = control-ref of="General trigger settings"() -> (w55:refnum<vi>)
  n23 = control-ref of="Trigger HW config"() -> (w54:refnum<vi>)
  n24 = control-ref of="XY stage available"() -> (w19:refnum<vi>)
  n25 = control-ref of="Y stage available"() -> (w4:refnum<vi>)
  n26 = control-ref of="Laser Power Control HW config"() -> (w28:refnum<vi>)
  n27 = control-ref of="Laser 1 config"() -> (w27:refnum<vi>)
  n28 = control-ref of="Max Allowed Trial Length [s]"() -> (w58:refnum<vi>)
  n29 = control-ref of="Initial Scan Resolution"() -> (w57:refnum<vi>)
  n30 = control-ref of="Initial Acceptance Angle [mrad]"() -> (w56:refnum<vi>)
  n31 = control-ref of="Initial Laser Wavelength [nm]"() -> (w16:refnum<vi>)
  n32 = control-ref of="Initial Dwell Time [us]"() -> (w15:refnum<vi>)
  n33 = control-ref of="PMT Voltage Lower Limit"() -> (w8:refnum<vi>)
  n34 = control-ref of="PMT Voltage Upper Limit"() -> (w7:refnum<vi>)
  n35 = control-ref of="Z stage available"() -> (w2:refnum<vi>)
  n36 = control-ref of="AOD Settings - distilled"() -> (w35:refnum<vi>)
  n37 = control-ref of="Prechirper 1 config"() -> (w26:refnum<vi>)
  n38 = control-ref of="Prechirper Constants"() -> (w23:refnum<vi>)
  n39 = control-ref of="XY Comms Config Cluster"() -> (w5:refnum<vi>)
  n40 = control-ref of="Y Comms Config Cluster"() -> (w3:refnum<vi>)
  n41 = control-ref of="Microscope ID"() -> (w62:refnum<vi>)
  n42 = control-ref of="Microscope Type"() -> (w61:refnum<vi>)
  n43 = control-ref of="Revision Number"() -> (w60:refnum<vi>)
  n44 = control-ref of="Triggers output setup"() -> (w29:refnum<vi>)
  n45 = control-ref of="Z Comms Config Cluster"() -> (w1:refnum<vi>)
  n46 = control-ref of="Laser Wavelength"() -> (w22:refnum<vi>)
  n47 = control-ref of="Pane"() -> (w72:refnum<vi>)
  n48 = control-ref of="XYZ Stage Control Config"() -> (w6:refnum<vi>)
  n49 = control-ref of="Encoder available"() -> (w46:refnum<vi>)
  n50 = control-ref of="Cam VidRec available"() -> (w36:refnum<vi>)
  n51 = control-ref of="Pockels cal.Zoom"() -> (w33:refnum<vi>)
  n52 = control-ref of="Pockels cal.Dwell time (µs)"() -> (w32:refnum<vi>)
  n53 = control-ref of="PreChirper Preset Calibration Values"() -> (w24:refnum<vi>)
  n54 = control-ref of="Encoder"() -> (w47:refnum<vi>)
  n55 = control-ref of="Current Objective"() -> (w31:refnum<vi>)
  n56 = control-ref of="Cam VidRec"() -> (w37:refnum<vi>)
  n57 = control-ref of="Encoder port"() -> (w45:refnum<vi>)
  n58 = control-ref of="Wheel radius (cm)"() -> (w43:refnum<vi>)
  n59 = control-ref of="Objective Calibration Settings"() -> (w30:refnum<vi>)
  n60 = control-ref of="Swap XY on stage"() -> (w41:refnum<vi>)
  n61 = control-ref of="Axial MC Supported"() -> (w39:refnum<vi>)
  n62 = control-ref of="MC Supported"() -> (w38:refnum<vi>)
  n63 = control-ref of="Encoder IP address"() -> (w44:refnum<vi>)
  n64 = control-ref of="Number of AODs"() -> (w40:refnum<vi>)
  n65 = call <userlib>:"Current VIs Reference__ogtk.vi"() -> ("Current VI's reference"=w67:refnum<vi>)  [unwired: 5 in]
  n66 = Current VI's Menubar() -> (w76:refnum<k9>)
  n67 = control-ref of="Demo mode"() -> (w42:refnum<vi>)
  n68 = control-ref of="Computer MAC address"() -> (w34:refnum<vi>)
  n69 = Bundle By Name(cluster=T29 {"VI's reference"=refnum, "menu reference"=refnum, "Pane"=refnum, "Config Tab Control"=refnum, "Triggers sub-tab control"=refnum, "Microscope ID"=refnum, "Microscope Type"=refnum, "Revision Number"=refnum, "Advanced Imaging"=refnum, "Max Allowed Trial Length"=refnum, "Initial Scan Resolution"=refnum, "Initial Acceptance Angle"=refnum, "Initial Laser Wavelength [nm] "=refnum, "Initial Dwell Time [us]"=refnum, "Error Logging"=refnum, "Performance Monitoring"=refnum, "Ctrl FPGA available"=refnum, "Control HW config"=refnum, "Control System Config"=refnum, "General trigger settings"=refnum, "Trigger HW config"=refnum, "Externalise Triggers"=refnum, "[Triggers output setup]"=refnum, "DAQ FPGA HW Config"=refnum, "DAQ FPGA System Config"=refnum, "Pockels AO"=refnum, "Hard shutter AO"=refnum, "PMT AOs"=refnum, "Galvo AO"=refnum, "Power meter AI"=refnum, "PMT Voltage Lower Limit"=refnum, "PMT Voltage Upper Limit"=refnum, "XYZ Stage Control Config"=refnum, "XY stage available"=refnum, "XY Comms Config Cluster"=refnum, "Y stage available"=refnum, "Y Comms Config Cluster"=refnum, "Z stage available"=refnum, "Z Comms Config Cluster"=refnum, "Encoder available"=refnum, "Encoder"=refnum, "Encoder IP address"=refnum, "Encoder port"=refnum, "Wheel radius (cm)"=refnum, "Demo mode"=refnum, "Swap XY on stage"=refnum, "Number of AODs"=refnum, "Axial MC Supported"=refnum, "MC Supported"=refnum, "Computer MAC add."=refnum, "Cam VidRec available"=refnum, "Cam VidRec"=refnum, "DO flag-Video record"=refnum, "DO flag-Trial start"=refnum, "AOD Settings (distilled)"=refnum, "Pockels cal.Dwell time (µs)"=refnum, "Pockels cal.Zoom"=refnum, "Current Objective"=refnum, "[Obj. Calib. Settings]"=refnum, "Laser Wavelength"=refnum, "Laser Power Control \nHW config"=refnum, "Laser 1 available"=refnum, "Laser 1 config"=refnum, "Prechirper 1 available"=refnum, "Prechirper 1 config"=refnum, "PreChirp Preset Values"=refnum, "[PreChirper Preset \nCalibration Values]"=refnum, "Prechirper Constants"=refnum} ("Pos ctrl window refs"), "VI's reference"=w67, "menu reference"=w76, "Pane"=w72, "Config Tab Control"=w21, "Triggers sub-tab control"=w63, "Microscope ID"=w62, "Microscope Type"=w61, "Revision Number"=w60, "Advanced Imaging"=w59, "Max Allowed Trial Length"=w58, "Initial Scan Resolution"=w57, "Initial Acceptance Angle"=w56, "Initial Laser Wavelength [nm]"=w16, "Initial Dwell Time [us]"=w15, "Error Logging"=w14, "Performance Monitoring"=w13, "Ctrl FPGA available"=w20, "Control HW config"=w12, "Control System Config"=w11, "General trigger settings"=w55, "Trigger HW config"=w54, "Externalise Triggers"=w53, "[Triggers output setup]"=w29, "DAQ FPGA HW Config"=w10, "DAQ FPGA System Config"=w9, "Pockels AO"=w52, "Hard shutter AO"=w51, "PMT AOs"=w50, "Galvo AO"=w49, "Power meter AI"=w48, "PMT Voltage Lower Limit"=w8, "PMT Voltage Upper Limit"=w7, "XYZ Stage Control Config"=w6, "XY stage available"=w19, "XY Comms Config Cluster"=w5, "Y stage available"=w4, "Y Comms Config Cluster"=w3, "Z stage available"=w2, "Z Comms Config Cluster"=w1, "Encoder"=w47, "Encoder available"=w46, "Encoder IP address"=w44, "Encoder port"=w45, "Wheel radius (cm)"=w43, "Demo mode"=w42, "Swap XY on stage"=w41, "Number of AODs"=w40, "Axial MC Supported"=w39, "MC Supported"=w38, "Computer MAC add."=w34, "Cam VidRec"=w37, "DO flag-Video record"=w71, "DO flag-Trial start"=w70, "Cam VidRec available"=w36, "AOD Settings (distilled)"=w35, "Pockels cal.Zoom"=w33, "Pockels cal.Dwell time (µs)"=w32, "Current Objective"=w31, "[Obj. Calib. Settings]"=w30, "Laser Wavelength"=w22, "Laser Power Control \nHW config"=w28, "Laser 1 available"=w18, "Laser 1 config"=w27, "Prechirper 1 available"=w17, "Prechirper 1 config"=w26, "PreChirp Preset Values"=w25, "[PreChirper Preset \nCalibration Values]"=w24, "Prechirper Constants"=w23) -> (w64:T29)
  n70 = call <vilib>:"Set Busy.vi"() -> ("error out"=w75:errorcluster)  [unwired: 10 in, 1 out]
  n71 = control-ref of="Objective Calibration Settings"() -> ()  [unwired: 1 out]
  n72 = call "Sys config window-Initialise.vi"("Disable positioning"=w68, "Window Name (i.e. Key)"=w69, "error in (no error)"=w75, "Pos ctrl window refs"=w64) -> ("error out"=w74:errorcluster, "output cluster"=w66:T30)  [unwired: 6 in]
  n73 = call <vilib>:"Unset Busy.vi"("error in (no error)"=w74) -> ("error out"=w73:errorcluster)  [unwired: 10 in]
  n74 = while {
    tunnel: w73 -> [w81]
    tunnel: w67 -> [w83]
    tunnel: [w83] -> w77
    tunnel: w66 -> [w80]
    tunnel: [w79] -> w65
    stop <- w79 stop-if-true
    n75 = event shown="[0] Timeout" {
      selector: _ -> [_ _ _ _ _ _]
      dyn-events: _ -> [_ _ _ _ _ _]
      timeout: 200 -> [_ _ _ _ _ _]
      tunnel: [w85 _ w103 _ w116 w117] -> w79
      tunnel: w81 -> [w86 _ _ _ _ _]
      tunnel: w80 -> [_ _ w101 _ w115 w118]
      event Timeout {
        n76 = event-data() -> ()  [unwired: 1 in, 1 out]
        n77 = case shown="Error" w86 {
          selector: w86 -> [_ w94]
          tunnel: [w92 w95] -> w85
          frame No Error {
            n78 = global read "General Globals.vi" "Stop application"() -> (w92:bool)
          }
          frame Error {
            w95 = TRUE  # Close
            n79 = call "Window-Error message.vi"("error in (no error)"=w94, "Message"="An error occured when initialising the System Configuration window.\nThe window will now close." ("Error Source")) -> ()  [unwired: 9 in, 1 out]
          }
        }
        n80 = global read "Sys Config window globals.vi" "Bring to front"() -> (w84:bool)
        n81 = case shown="True" w84 {
          frame False {
          }
          frame True {
            n82 = call <userlib>:"Current VIs Reference__ogtk.vi"() -> ("Current VI's reference"=w91:refnum<vi>)  [unwired: 5 in]
            n83 = property class="VI"(reference=w91, "Front Panel.IsFrontmost"=TRUE ("Front Panel Window:Is Frontmost"), "FP.State"=T38."Standard" ("Front Panel Window:State")) -> (reference out=w90:refnum<vi>)  [unwired: 1 in, 1 out]
            n84 = global write "Sys Config window globals.vi" "Bring to front"(FALSE ("Bring to front")) -> ()
            n85 = Close Reference(reference=w90) -> ()  [unwired: 1 in, 1 out]
          }
        }
      }
      event "Externalise Triggers", "Encoder available", "Cam VidRec available", "MC Supported": Value Change {
        # "Handles the top level window's UI"
        # "Handles the top level window's UI"
        # "Handles this window's UI"
        # "When this code executes it sets the \"Enabled\" state of Video Recording related UI elements throughout the software, depending on the \"VidRec available\" parameter's setting. The setting is not changed in the FGV until later when the \"OK\" button is pressed. This code here offers just a \"live preview\" of the effect this setting has on the UI."
        n86 = event-data() -> ()  [unwired: 1 in, 1 out]
        n87 = call "Set Encoder UI from file.vi"("Encoder available"="Encoder available") -> ()  [unwired: 10 in, 1 out]
        n88 = call "Enable-Disable Encoder UI.vi"("Cam VidRec.VidRec available"="Encoder available") -> ()  [unwired: 10 in, 1 out]
        n89 = call "Sys config window-Set disabled states.vi"() -> ()  [unwired: 11 in, 1 out]
        n90 = call "Enable-Disable MovCor UI.vi"("MC Supported"="MC Supported") -> ()  [unwired: 11 in]
        n91 = call "Enable-Disable VidRec UI.vi"("Cam VidRec.VidRec available"="Cam VidRec available") -> ()  [unwired: 10 in, 1 out]
      }
      event "OK": Value Change {
        # ">>Initial config >>"
        n92 = event-data() -> ()  [unwired: 1 in, 1 out]
        n93 = call "Sys config window-Get set control values.vi"("Function"=Get-Set-Clear_Control."Get") -> ("output cluster"=w100:T30)  [unwired: 9 in, 1 out]
        n94 = Not Equal?(x=w101, y=w100) -> (x != y?=w99:bool)
        n95 = case shown="True" w99 {
          tunnel: [TRUE w106] -> w103
          tunnel: w101 -> [_ w105]
          frame False {
          }
          frame True {
            n96 = call "Sys config window-Check valid setup.vi"() -> ("Continue"=w107:bool)  [unwired: 11 in]
            n97 = case shown="True" w107 {
              tunnel: [FALSE TRUE] -> w106
              tunnel: w105 -> [_ w109]
              frame False {
              }
              frame True {
                n98 = disable-structure shown="Disabled" {
                  disable-tunnel: w109 -> [w111 _]
                  frame Disabled {
                    n99 = call "Sys config window-Save HW config.vi"("Initial Configuration"=w111) -> ()  [unwired: 11 in]
                  }
                  frame Enabled {
                  }
                }
                n100 = call "Sys config-process changes.vi"("Initial Configuration"=w109) -> ()  [unwired: 11 in]
              }
            }
          }
        }
      }
      event Value Change {
        w113 = 6  # Limited to 6 triggers
        # "May be upgraded in the future to handle more. The triggers functionality already uses an array provisionally."
        n101 = event-data() -> ("NewVal"=w114:T17)  [unwired: 1 in, 5 out]
        n102 = Array Subset(array=w114, length=w113) -> (w112:T17)  [unwired: 1 in]
        n103 = local write "Triggers output setup"(w112) -> ()
      }
      event "Cancel": Value Change {
        n104 = event-data() -> ()  [unwired: 1 in, 1 out]
        n105 = call "Sys config window-Exit dialogue.vi"("Initial Configuration"=w115) -> ("Close"=w116:bool)  [unwired: 10 in]
      }
      event Panel Close? {
        n106 = event-data() -> ()  [unwired: 1 in, 1 out]
        n107 = call "Sys config window-Exit dialogue.vi"("Initial Configuration"=w118) -> ("Close"=w117:bool)  [unwired: 10 in]
        n108 = Not(x=w117) -> (.not. x?=w119:bool)
        n109 = event-data("Discard?"=w119) -> ()  [unwired: 1 in, 1 out]
      }
    }
  }
  n110 = control-ref of="Control system"() -> ()  [unwired: 1 out]
  n111 = flat-sequence {
    tunnel: w77 -> [w123]
    tunnel: w69 -> [w121]
    frame #0 {
      n112 = global write "Sys Config window globals.vi" "Window is open"(FALSE ("Bring to front")) -> ()
      n113 = call "Save_Windows_Bounds.vi"("Window Name (i.e. Key)"=w121, "Front Panel Window:Open"=FALSE, "Window VI's Ref"=w123) -> ()  [unwired: 8 in, 1 out]
    }
  }
  n114 = flat-sequence {
    tunnel: w65 -> [_]
    frame #0 {
      n115 = global read "gl_UI Ctrl Refs.vi" "UI ctrl refs"() -> (w126:T41)
      n116 = call "fgv_Sys and HW Config.vi"("Function"=HW_config_states_enum."Read all") -> ("Hardware Configuration OUT"=w124:T32)  [unwired: 8 in, 2 out]
      n117 = Unbundle By Name(w124) -> ("Encoder available"=w125:bool)
      n118 = Unbundle By Name(w126) -> ("Speed Logging"=w127:refnum<vi>)
      n119 = Unbundle By Name(w124) -> ("VidRec available"=w129:bool)
      n120 = Unbundle By Name(w124) -> ("MC Supported"=w130:bool)
      n121 = property class="Bool (strict)"(reference=w127, "Value"=w125) -> ()  [unwired: 1 in, 2 out]
      n122 = call "Enable-Disable VidRec UI.vi"("Cam VidRec.VidRec available"=w129) -> ()  [unwired: 10 in, 1 out]
      n123 = call "Enable-Disable MovCor UI.vi"("MC Supported"=w130) -> ()  [unwired: 11 in]
      n124 = call "Enable-Disable Encoder UI conditionally.vi"() -> ()  [unwired: 11 in, 1 out]
    }
  }
